vi "new counter entry.vi"(8 "error in":errorcluster, 11 "Small?":bool) -> (0 "error out":errorcluster, 3 "Integer Time":i64)   [LabVIEW 2013]
doc: "Creates a new row in the counter or counter_small table."
uses:
  <vilib>/addons/database/NI_Database_API.lvlib
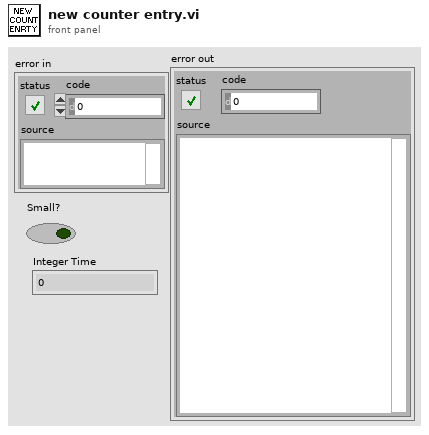
[diagram p1: front panel]
types:
  T1 = typedef "NI_Database_API.lvlib/Conn ObjectReference.ctl" = refnum<k1>
  T2 = cluster{"Integer Timestamp":i64, "Integer Time":i64, "Integer Timestamp":i64, "Integer Timestamp":i64, "Integer Timestamp":i64, "Integer Timestamp":i64}
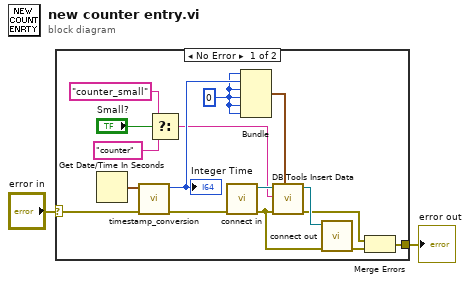
[diagram p0: block diagram]
diagram:
  n1 = case shown="No Error" "error in" {
    selector: "error in" -> [w8 w19]
    tunnel: [w18 w19] -> w1
    frame No Error {
      w7 = i64 0 ("Integer Timestamp")
      n2 = Get Date/Time In Seconds() -> (seconds since 1Jan1904=w17:timestamp)
      n3 = call "timestamp_conversion.vi"("error in (no error)"=w8, "Time Stamp"=w17) -> ("error out"=w9:errorcluster, "Integer Time"=w16:i64)  [unwired: 7 in]
      "Integer Time" <- w16
      n4 = Select(t="counter_small", s="Small?", f="counter" ("table")) -> (s? t:f=w4:string)
      n5 = call "connect in.vi"("error in (no error)"=w9) -> ("error out"=w12:errorcluster, "Database Connection"=w15:T1)  [unwired: 6 in, 1 out]
      n6 = Bundle("Integer Timestamp"=w7, "Integer Time"=w16, "Integer Timestamp"=w7, "Integer Timestamp"=w7, "Integer Timestamp"=w7, "Integer Timestamp"=w7) -> (w10:T2)  [unwired: 1 in]
      n7 = call <vilib>:"DB Tools Insert Data.vi"("data"=w10, "error in (no error)"=w12, "table"=w4, "connection reference"=w15) -> ("error out"=w13:errorcluster, "connection reference out"=w14:T1)  [unwired: 6 in]
      n8 = call "connect out.vi"("error in (no error)"=w12, "connection reference"=w14) -> ("error out"=w11:errorcluster)  [unwired: 9 in]
      n9 = Merge Errors(w13, w11) -> (w18:errorcluster)
    }
    frame Error {
    }
  }
  "error out" <- w1
